vi "Variables_locales.vi"() -> ()   [LabVIEW 2020]
panel:
  out "Boolean 2":bool
  in  "stop":bool
  out "Waveform Chart 2":dbl(graph)
  out "Waveform Chart":dbl(graph)
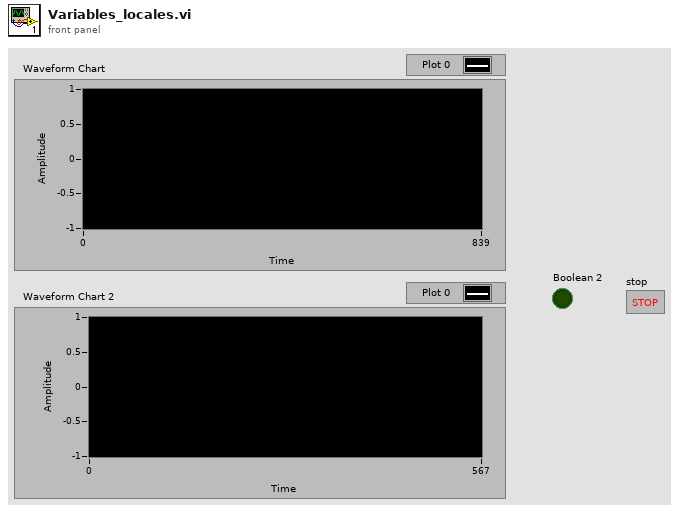
[diagram p1: front panel]
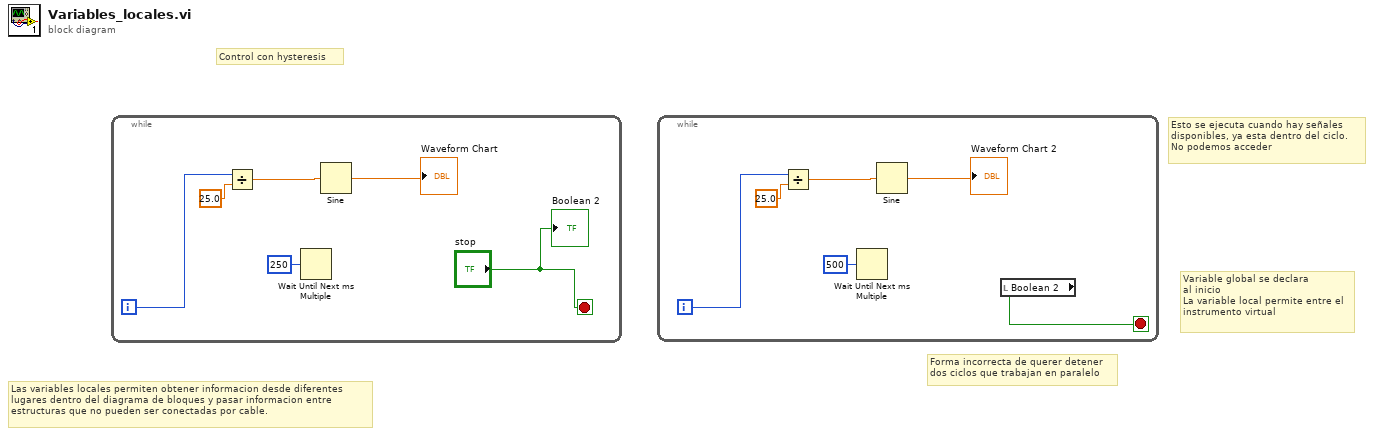
[diagram p0: block diagram]
diagram:
  # "Las variables locales permiten obtener informacion desde diferentes \nlugares dentro del diagrama de bloques y pasar informacion entre \nestructuras que no pueden ser conectadas por cable."
  # "Variable global se declara\nal inicio\nLa variable local permite entre el\ninstrumento virtual"
  # "Forma incorrecta de querer detener\ndos ciclos que trabajan en paralelo"
  # "Esto se ejecuta cuando hay señales \ndisponibles, ya esta dentro del ciclo. \nNo podemos acceder"
  # "Control con hysteresis"
  n1 = while {
    i -> [w5]
    stop <- "stop" stop-if-true
    n2 = Divide(x=w5, y=25.0) -> (x/y=w4:dbl)
    n3 = Wait Until Next ms Multiple(millisecond multiple=u32 250) -> ()  [unwired: 1 out]
    n4 = Sine(x=w4) -> (sin(x)=→"Waveform Chart":dbl)
    "Boolean 2" <- "stop"
  }
  n5 = while {
    i -> [w11]
    stop <- w7 stop-if-true
    n6 = Divide(x=w11, y=25.0) -> (x/y=w10:dbl)
    n7 = Wait Until Next ms Multiple(millisecond multiple=u32 500) -> ()  [unwired: 1 out]
    n8 = Sine(x=w10) -> (sin(x)=→"Waveform Chart 2":dbl)
    n9 = local read "Boolean 2"() -> (w7:bool)
  }
